vi "NI6602.Reset Integral Values.vi"(0 "i ref in":refnum<vi>, 5 "error in (no error)":errorcluster) -> (14 "i ref out":refnum<vi>, 19 "error out":errorcluster)   [LabVIEW 2014, in "NI6602.lvlib"]
doc: "Resets the integral values to 0.\n\nLicense Agreement for this software:\n\nCopyright (C)\nGesellschaft für Schwerionenforschung, GSI\nPlanckstr. 1\n64291 Darmstadt\nGermany\n\nContact: D.Beck@gsi.de \n\nThis program is free software; you can redistribute it and/or modify it under the terms of the \nGNU General Public License as published by the Free Software Foundation; either version 2 of \nthe license, or (at your option) any later version.\n\nThis program is distributed in the hope that it will be useful, but WITHOUT ANY WARRANTY; \nwithout even the implied warranty of MERCHANTABILITY or FITNESS FOR A PARTICULAR PURPOSE. See the GNU General License for more details (http://www.gnu.org).\n\nGesellschaft für Schwerionenforschung, GSI\nPlanckstr. 1, 64291 Darmstadt, Germany\nFor all questions and ideas contact: M.Richter@gsi.de, H.Brand@gsi.de or D.Beck@gsi.de.\nLast update: 16-JUN-2004"
uses:
  NI6602.lvlib
  CSlibraries-extern/DimLVEvent/LVDimInterface/LVDimInterface.lvlib
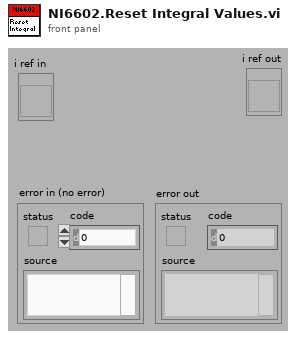
[diagram p1: front panel]
types:
  T1 = typedef "NI6602.lvlib/NI6602.i attribute.ctl" = cluster{"CounterDAQ Channels":cluster{"task":refnum<k21>, "Channel Name":string}[], "RateServiceIDs":i32[], "Running?":bool, "IntegralServiceIDs":i32[], "ThresholdID":i32, "Threshold":dbl, "IntegralValues":dbl[], "Stopped?":bool}
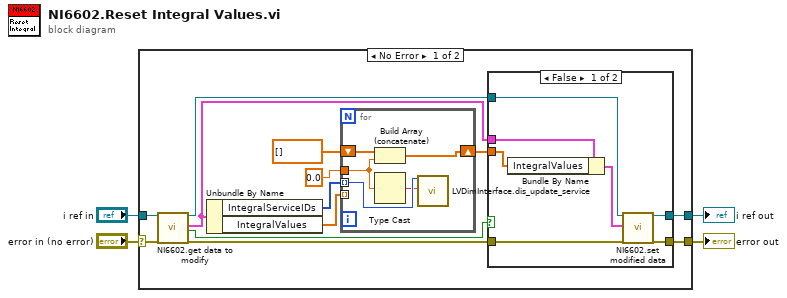
[diagram p0: block diagram]
diagram:
  n1 = case shown="No Error" "error in (no error)" {
    selector: "error in (no error)" -> [w16 w33]
    tunnel: [w12 w32] -> w4
    tunnel: [w11 w33] -> w3
    tunnel: "i ref in" -> [w17 w32]
    frame No Error {
      n2 = call "NI6602.get data to modify.vi"("i ref in"=w17, "error in (no error)"=w16) -> ("i ref out"=w14:refnum<vi>, "i attribute"=w10:T1, "timed out"=w15:bool, "error out"=w13:errorcluster)  [unwired: 14 in]
      n3 = Unbundle By Name(w10) -> ("IntegralServiceIDs"=w5:i32[], "IntegralValues"=w9:dbl[])
      n4 = for {
        tunnel: w9 -> [_] mode=indexing
        shift-right: [w21] -> w6
        shift-left: dbl[] [] ("IntegralValues") -> [w22]
        tunnel: 0.0 ("my_serviceID") -> [w18]
        tunnel: w5 -> [w20] mode=indexing
        n5 = Build Array (concatenate)(w22, w18) -> (w21:dbl[])
        n6 = Type Cast(x=w18) -> (*(type *) &x=w19:string)  [unwired: 1 in]
        n7 = call "LVDimInterface.dis_update_service.vi"("my_serviceID"=w20, "data"=w19) -> ()  [unwired: 15 in, 3 out]
      }
      n8 = case shown="False" w15 {
        tunnel: w14 -> [w29 w31]
        tunnel: w13 -> [w28 w30]
        tunnel: [w27 w31] -> w12
        tunnel: [w26 w30] -> w11
        tunnel: w10 -> [w25 _]
        tunnel: w6 -> [w23 _]
        frame False {
          n9 = Bundle By Name(cluster=w25, "IntegralValues"=w23) -> (w24:T1)
          n10 = call "NI6602.set modified data.vi"("i ref in"=w29, "i attribute"=w24, "error in (no error)"=w28) -> ("i ref out"=w27:refnum<vi>, "error out"=w26:errorcluster)  [unwired: 15 in]
        }
        frame True {
        }
      }
    }
    frame Error {
    }
  }
  "i ref out" <- w4
  "error out" <- w3
